vi "IsConnect LTS Stage.vi"(8 "error in (no error)":errorcluster, 10 "Cluster in":T1, 11 "LTS Reference In":refnum<k24>) -> (0 "error out":errorcluster, 1 "IsConnected":bool, 2 "Cluster out":T1, 3 "LTS Reference Out":refnum<k24>)   [LabVIEW 2018]
uses:
  Controls/Translation Stage Cluster.ctl
  General/Controls/Translation Stage Types.ctl
  C:/Project/SerialSectionOCT/SerialSectOCT/Labview Software/Thorlabs.MotionControl.Controls.dll
  Thorlabs.MotionControl.Controls.dll
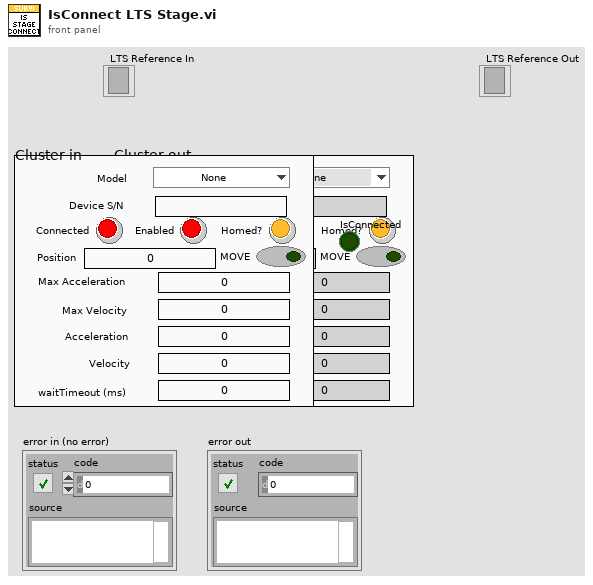
[diagram p1: front panel]
types:
  T1 = typedef "Translation Stage Cluster.ctl" = cluster{"Position":dbl, "Is.Enabled?":bool, "Is.Connected?":bool, "Device SN":string, "AccelerationMaximum":dbl, "VelocityMaximum":dbl, "Acceleration":dbl, "Velocity":dbl, "waitTimeout (ms)":i32, "Model":T2, "Is.Homed?":bool, "MOVE":bool}
  T2 = typedef "Translation Stage Types.ctl" = enum16{"None", "Thorlabs LTS", "Thorlabs MLJ"}
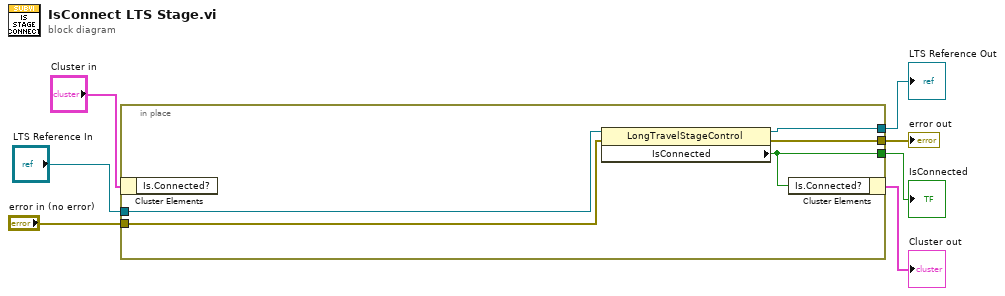
[diagram p0: block diagram]
diagram:
  n1 = in-place {
    in-place-border: "LTS Reference In" -> [w8]
    in-place-border: [w12] -> w5
    in-place-border: "error in (no error)" -> [w9]
    in-place-border: [w11] -> w3
    in-place-border: [w10] -> w1
    n2 = in-place-cluster #1("Cluster in") -> ()  [unwired: 1 out]
    n3 = property class="LongTravelStageControl"(reference=w8, error in=w9) -> (reference out=w12:refnum<k24>, error out=w11:errorcluster, "IsConnected"=w10:bool)
    n4 = in-place-cluster #1("Is.Connected?"=w10) -> (→"Cluster out":T1)
  }
  "error out" <- w3
  "LTS Reference Out" <- w5
  "IsConnected" <- w1
